vi "Read Digitals (Batch).vi"(0 "connection ID":refnum<k16>, 1 "address":u32, 2 "port":u16, 9 "timeout ms (1000)":i32=1000, 11 "error in (no error)":errorcluster) -> (4 "connection ID out":refnum<k16>, 6 "received data":string, 8 "Digitals":bool[](array[boolean]), 15 "error out":errorcluster)   [LabVIEW 2016, in "instr.lvlib"]
doc: "Reads all digital states and returns them as array. Batch operation."
uses:
  instr.lvlib
  IO State.ctl
panel:
  out "Send String":string
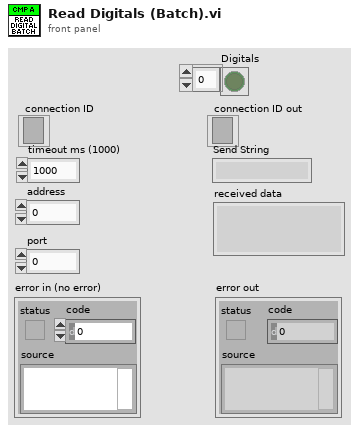
[diagram p1: front panel]
types:
  T1 = typedef "instr.lvlib/IO State.ctl" = u16
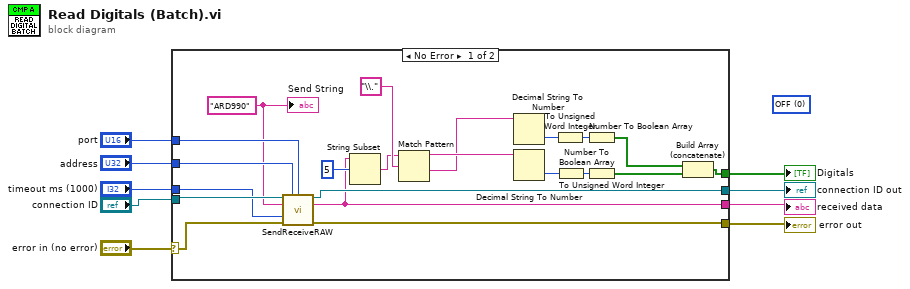
[diagram p0: block diagram]
diagram:
  (unwired) T1 0 items=["OFF", "ON"] ("Relay State")
  n1 = case shown="No Error" "error in (no error)" {
    selector: "error in (no error)" -> [w10 w32]
    tunnel: [w30 w32] -> w9
    tunnel: "timeout ms (1000)" -> [w27 _]
    tunnel: "connection ID" -> [w28 w31]
    tunnel: [w29 w31] -> w5
    tunnel: "address" -> [w26 _]
    tunnel: "port" -> [w25 _]
    tunnel: [w22 _] -> w2
    tunnel: [w20 _] -> w1
    frame No Error {
      w24 = "ARD990" ("data in")
      n2 = call "SendReceiveRAW.vi"("connection ID"=w28, "address"=w26, "port"=w25, "RAW data in"=w24, "timeout ms (1000)"=w27, "error in (no error)"=w10) -> ("connection ID out"=w29:refnum<k16>, "received data"=w22:string, "error out"=w30:errorcluster)  [unwired: 7 in]
      n3 = String Subset(string=w22, offset (0)=5 ("offset")) -> (substring=w13:string)  [unwired: 1 in]
      n4 = Match Pattern(string=w13, regular expression="\\.") -> (before substring=w12:string, after substring=w11:string)  [unwired: 1 in, 2 out]
      n5 = Decimal String To Number(string=w11) -> (number=w17:i32)  [unwired: 2 in, 1 out]
      n6 = Decimal String To Number(string=w12) -> (number=w18:i32)  [unwired: 2 in, 1 out]
      n7 = To Unsigned Word Integer(number=w17) -> (unsigned 16bit integer=w16:u16)
      n8 = To Unsigned Word Integer(number=w18) -> (unsigned 16bit integer=w19:u16)
      n9 = Number To Boolean Array(number=w16) -> (Boolean array=w15:bool[])
      n10 = Number To Boolean Array(number=w19) -> (Boolean array=w14:bool[])
      n11 = Build Array (concatenate)(w15, w14) -> (w20:bool[])
      "Send String" <- w24
    }
    frame Error {
    }
  }
  "error out" <- w9
  "received data" <- w2
  "connection ID out" <- w5
  "Digitals" <- w1
